vi "arreglos.vi"() -> ()   [LabVIEW 2020]
uses:
  53ed5e52-afaa-41b1-8cc3-f30a431db702.vi
  7dd8f612-86f7-495f-b1d8-28f3b0f895d0.vi
panel:
  out "array out 2":dbl[](array[numeric])
  out "array out":dbl[](array[numeric])
  out "index of element":i32
  out "min index(es)":i32
  out "min value":dbl
  out "max index(es)":i32
  out "max value":dbl
  out "appended array":dbl[](array[numeric])
  in  "Numeric 4":dbl
  in  "Numeric 3":dbl
  in  "Numeric 2":dbl
  in  "Numeric":dbl
  out "initialized array 2":bool[](array[boolean])
  out "initialized array":dbl[](array[numeric])
  out "subarray":u16[](array[numeric])
  out "output array 2":u16[](array[numeric])
  in  "nivel del tanque":u16(slide) scale=0.0..10.0
  in  "Velocimetro":u16(knob) scale=0.0..10.0
  out "size(s)":i32
  out "element 4":string
  out "output array":bool[](array[boolean])
  out "element 3":dbl
  out "element 2":dbl
  out "element":dbl
  in  "Array 4":u16[](array[numeric])
  in  "Array 3":string[](array[string])
  in  "Array 2":bool[](array[boolean])
  in  "Array":dbl[](array[slide]) scale=0.0..100.0
  # "Arreglos"
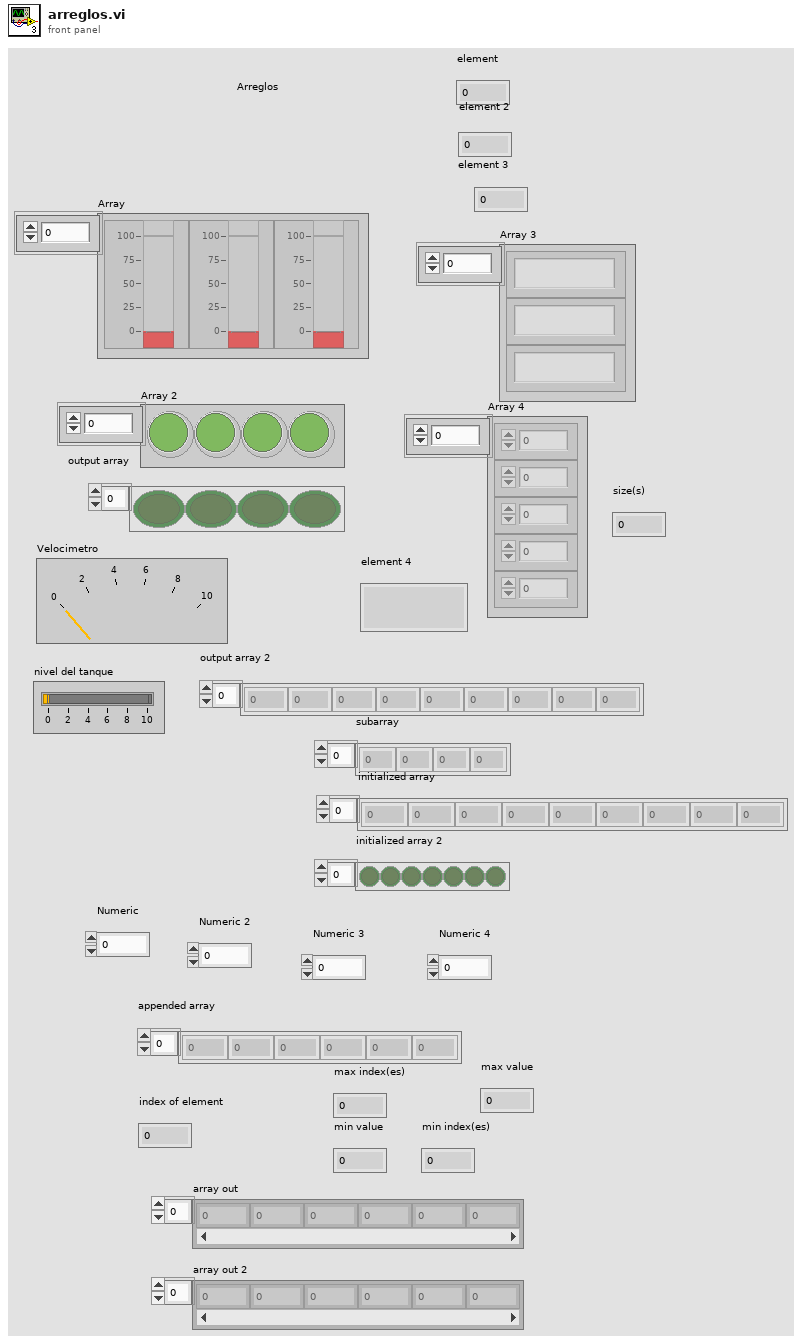
[diagram p1: front panel]
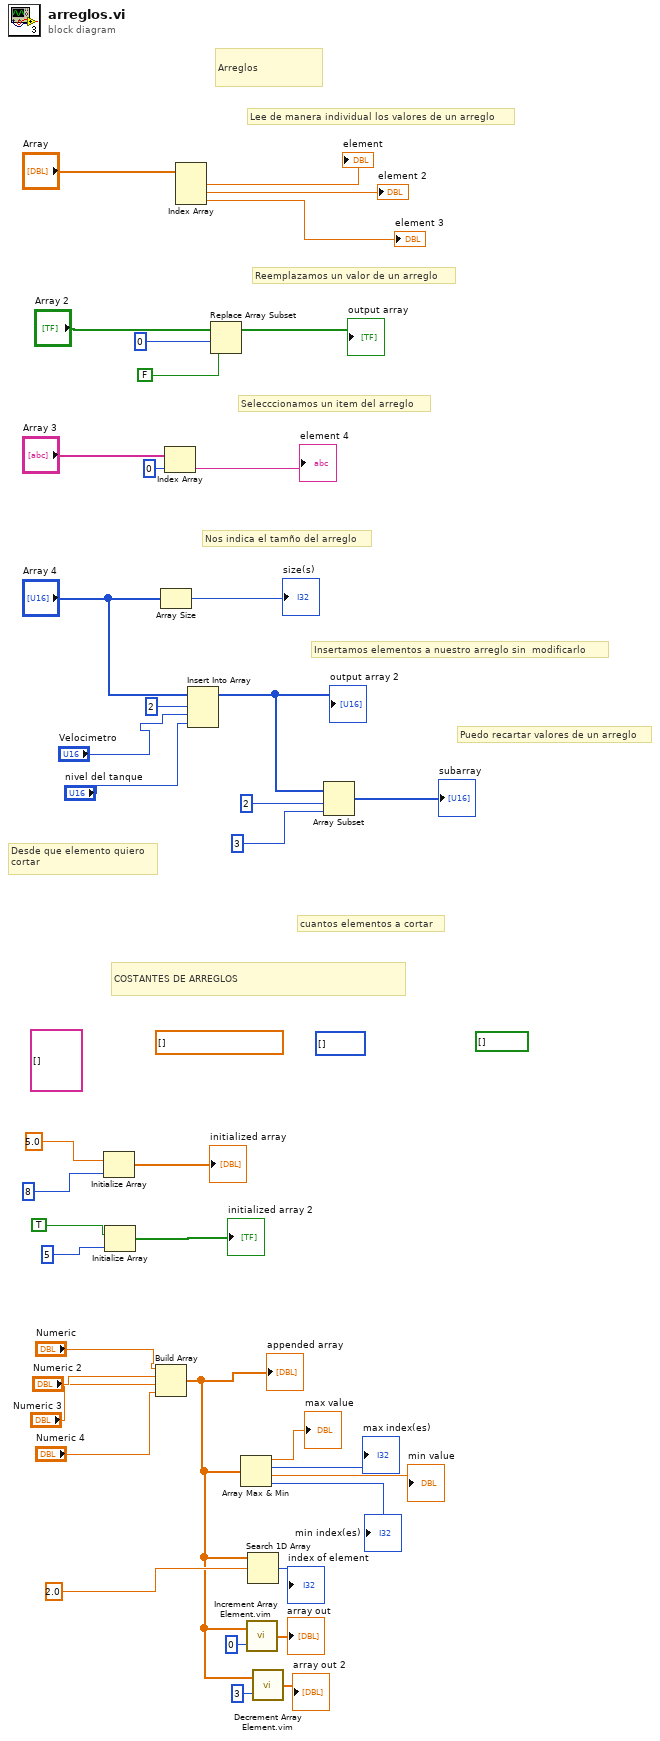
[diagram p0: block diagram]
diagram:
  (unwired) bool[] []
  (unwired) i32[] []
  (unwired) dbl[] []
  (unwired) string[] []
  # "COSTANTES DE ARREGLOS"
  # "Puedo recartar valores de un arreglo"
  # "cuantos elementos a cortar"
  # "Desde que elemento quiero\ncortar"
  # "Insertamos elementos a nuestro arreglo sin  modificarlo"
  # "Nos indica el tamño del arreglo"
  # "Selecccionamos un item del arreglo"
  # "Reemplazamos un valor de un arreglo"
  # "Lee de manera individual los valores de un arreglo"
  # "Arreglos"
  n1 = Initialize Array(5.0 ("element"), 8 ("dimension size")) -> (→"initialized array":dbl[])
  n2 = Initialize Array(TRUE, 5 ("dimension size")) -> (→"initialized array 2":bool[])
  n3 = Build Array("Numeric", "Numeric 2", "Numeric 3", "Numeric 4") -> (w5:dbl[])
  "appended array" <- w5
  n4 = Array Size(array="Array 4") -> (size(s)=→"size(s)":i32)
  n5 = Index Array(array="Array 3", index=0) -> (element=→"element 4":string)
  n6 = Index Array(array="Array") -> (element #1=→"element":dbl, element #2=→"element 2":dbl, element #3=→"element 3":dbl)  [unwired: 3 in]
  n7 = Insert Into Array(array="Array 4", index=2, new element #1="Velocimetro", new element #2="nivel del tanque") -> (w25:u16[])
  "output array 2" <- w25
  n8 = Replace Array Subset(array="Array 2", new element=FALSE, index=0) -> (→"output array":bool[])
  n9 = Array Max & Min(array=w5) -> (max value=→"max value":dbl, max index (indices)=→"max index(es)":i32, min value=→"min value":dbl, min index (indices)=→"min index(es)":i32)
  n10 = call "Increment Array Element.vim"("index"=0, "array in"=w5) -> ("array out"=→"array out":dbl[])
  n11 = Search 1D Array(1D array=w5, element=2.0) -> (index of element=→"index of element":i32)  [unwired: 1 in]
  n12 = call "Decrement Array Element.vim"("index"=3, "array in"=w5) -> ("array out"=→"array out 2":dbl[])
  n13 = Array Subset(array=w25, index=2, length=3) -> (→"subarray":u16[])
